vi "Configure Average.vi"(7 "Average On (F)":bool, 8 "error in (no error)":errorcluster, 10 "Average":u32, 11 "SA-FSW in":refnum<class "SA-FSW.lvclass">) -> (0 "error out":errorcluster, 3 "SA-FSW out":refnum<class "SA-FSW.lvclass">)   [LabVIEW 2020, in "SA-FSW.lvclass"]
uses:
  SA-FSW.lvclass
  C:/Sandbox/RF Bench/Source Code/WiSpry Test Framework/Instruments/Spectrum Analyzer/Spectrum Analyzer.lvclass
  C:/Sandbox/RF Bench/Source Code/WiSpry Test Framework/Instruments/Instrument.lvclass
  Spectrum Analyzer.lvclass/Spectrum Analyzer.ctl
  Instrument.lvclass/Instrument.ctl
  Instrument.lvclass
  Spectrum Analyzer.lvclass
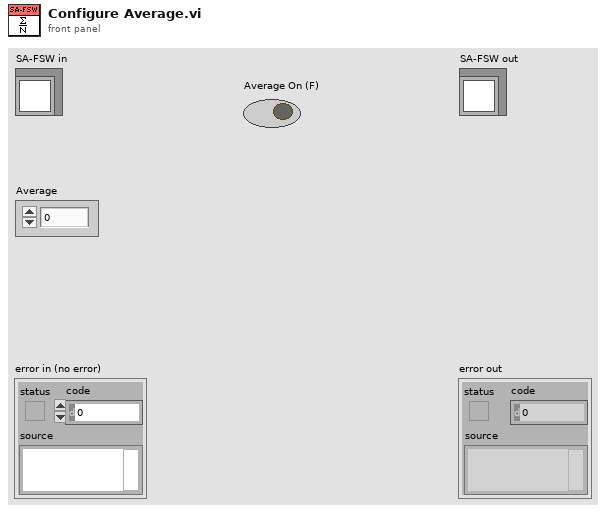
[diagram p1: front panel]
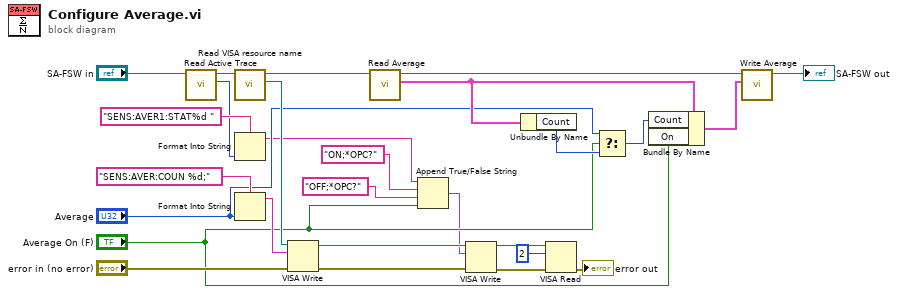
[diagram p0: block diagram]
diagram:
  n1 = call "Read Active Trace.vi"("Spectrum Analyzer in"="SA-FSW in") -> ("Active Trace"=w26:u16, "Spectrum Analyzer out"=w24:refnum<class "SA-FSW.lvclass">)  [unwired: 9 in]
  n2 = call "Read VISA resource name.vi"("Instrument in"=w24) -> ("VISA resource name"=w22:refnum<visa-resource-name>, "Instrument out"=w20:refnum<class "SA-FSW.lvclass">)  [unwired: 9 in]
  n3 = Format Into String(format string="SENS:AVER1:STAT%d " ("string (\"\")"), w26) -> (resulting string=w5:string)  [unwired: 2 in, 1 out]
  n4 = Format Into String(format string="SENS:AVER:COUN %d;", "Average") -> (resulting string=w6:string)  [unwired: 2 in, 1 out]
  n5 = VISA Write(VISA resource name=w22, write buffer=w6, error in (no error)="error in (no error)") -> (VISA resource name out=w11:refnum<visa-resource-name>, error out=w12:errorcluster)  [unwired: 1 out]
  n6 = call "Read Average.vi"("Spectrum Analyzer in"=w20) -> ("Average"=w17:cluster{"Count":u32, "On":bool}, "Spectrum Analyzer out"=w19:refnum<class "SA-FSW.lvclass">)  [unwired: 9 in]
  n7 = Append True/False String(1:"Average On (F)", 2:"OFF;*OPC?" ("false string"), 3:"ON;*OPC?" ("true string"), 4:w5) -> (0:w1:string)
  n8 = VISA Write(VISA resource name=w11, write buffer=w1, error in (no error)=w12) -> (VISA resource name out=w9:refnum<visa-resource-name>, error out=w10:errorcluster)  [unwired: 1 out]
  n9 = Unbundle By Name(w17) -> ("Count"=w15:u32)
  n10 = VISA Read(VISA resource name=w9, byte count=u32 2, error in (no error)=w10) -> (error out=→"error out":errorcluster)  [unwired: 3 out]
  n11 = Select(t="Average", s="Average On (F)", f=w15) -> (s? t:f=w14:u32)
  n12 = Bundle By Name(cluster=w17, "Count"=w14, "On"="Average On (F)") -> (w13:cluster{"Count":u32, "On":bool})
  n13 = call "Write Average.vi"("Average"=w13, "Spectrum Analyzer in"=w19) -> ("Spectrum Analyzer out"=→"SA-FSW out":refnum<class "SA-FSW.lvclass">)  [unwired: 9 in]
